vi "Lock Displays AE.vi"(0 "Lock All Markers":bool, 2 "Action":T1, 7 "Lock All AutoScale":bool, 11 "Lock Pan/Zoom":bool) -> (4 "Lock All Markers Out":bool, 8 "Lock All AutoScale Out":bool, 15 "Lock Pan/Zoom Out":bool)   [LabVIEW 2020]
uses:
  Hardware Configuration/Hardware Configuration Controls/Standard Action.ctl
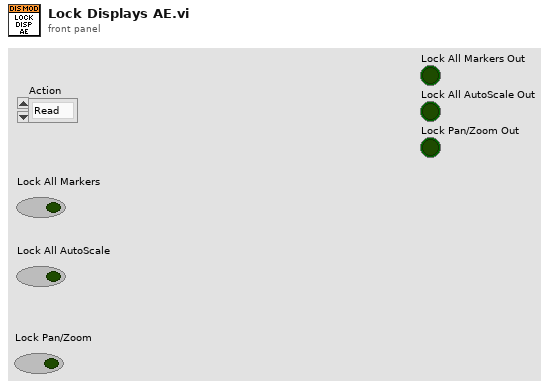
[diagram p1: front panel]
types:
  T1 = typedef "Standard Action.ctl" = enum16{"Read", "Write"}
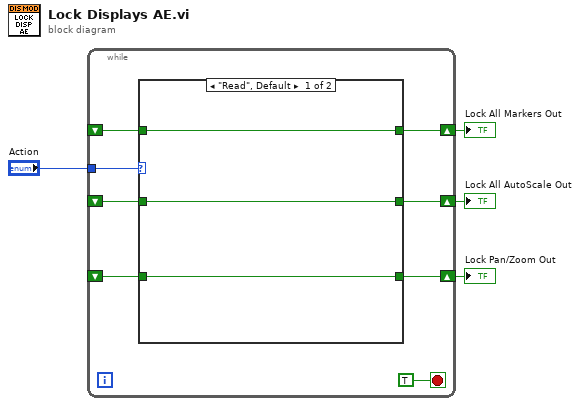
[diagram p0: block diagram]
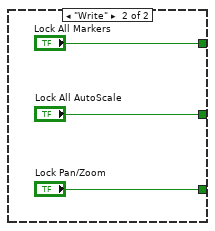
[diagram p2: hidden frame]
diagram:
  n1 = while {
    shift-right: [w10] -> w3
    shift-left: _ -> [w7]
    shift-right: [w9] -> w2
    shift-left: _ -> [w6]
    shift-right: [w8] -> w1
    shift-left: _ -> [w5]
    tunnel: "Action" -> [w11]
    stop <- TRUE stop-if-true
    n2 = case shown="\"Read\", Default" w11 {
      tunnel: [w15 "Lock All Markers"] -> w10
      tunnel: [w14 "Lock All AutoScale"] -> w9
      tunnel: [w13 "Lock Pan/Zoom"] -> w8
      tunnel: w7 -> [w15 _]
      tunnel: w6 -> [w14 _]
      tunnel: w5 -> [w13 _]
      frame "Read", Default {
      }
      frame "Write" {
      }
    }
  }
  "Lock All Markers Out" <- w3
  "Lock All AutoScale Out" <- w2
  "Lock Pan/Zoom Out" <- w1
